vi "Trap cluster 2 ROI.vi"(1 "Switch X/Y":bool, 2 "Trap cluster":T2, 3 "ROI in":T1) -> (0 "ROI out":T1)   [LabVIEW 2012]
uses:
  Trap cluster.ctl
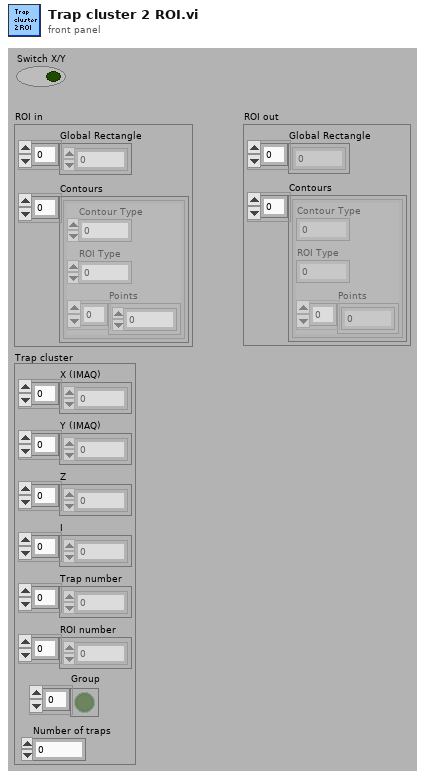
[diagram p1: front panel]
types:
  T1 = cluster{"Global Rectangle":i32[], "Contours":cluster{"Contour Type":u32, "ROI Type":u32, "Points":i32[]}[]}
  T2 = typedef "Trap cluster.ctl" = cluster{"X (IMAQ)":sgl[], "Y (IMAQ)":sgl[], "Z":sgl[], "I":sgl[], "Trap number":i32[], "ROI number":i32[], "Number of traps":i32, "Group":bool[]}
  T3 = cluster{"Contour Type":u32, "ROI Type":u32, "Points":i32[]}[]
  T4 = cluster{"Contour Type":u32, "ROI Type":u32, "Points":i32[]}
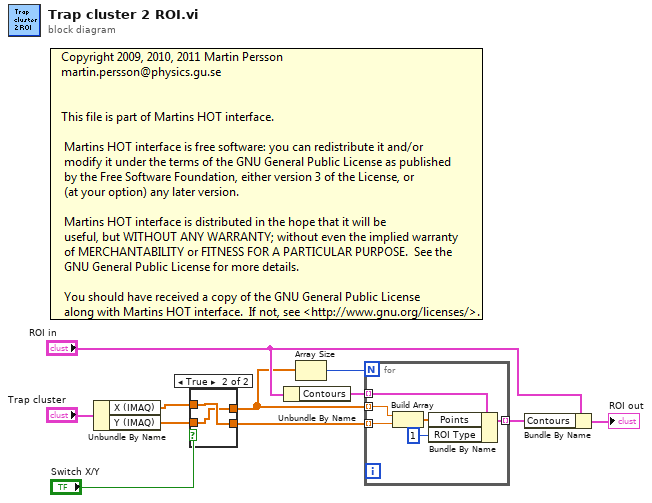
[diagram p0: block diagram]
diagram:
  n1 = Unbundle By Name("Trap cluster") -> ("X (IMAQ)"=w5:sgl[], "Y (IMAQ)"=w4:sgl[])
  n2 = case shown="True" "Switch X/Y" {
    tunnel: w5 -> [w13 w15]
    tunnel: [w12 w15] -> w3
    tunnel: w4 -> [w12 w14]
    tunnel: [w13 w14] -> w2
    frame False {
    }
    frame True {
    }
  }
  n3 = Unbundle By Name("ROI in") -> ("Contours"=w10:T3)
  n4 = Array Size(array=w2) -> (size(s)=w6:i32)
  n5 = for {
    N: w6 -> [_]
    tunnel: w2 -> [w21] mode=indexing
    tunnel: w3 -> [w20] mode=indexing
    tunnel: w10 -> [w19] mode=indexing
    tunnel: [w17] -> w11 mode=indexing
    n6 = Build Array(w21, w20) -> (w18:sgl[])
    n7 = Bundle By Name(cluster=w19, "Points"=w18, "ROI Type"=u32 1) -> (w17:T4)
  }
  n8 = Bundle By Name(cluster="ROI in", "Contours"=w11) -> (→"ROI out":T1)
